vi "String add from start.vi"(4 "Datetime Format":enum16{"Full", "HH:MM:SS"}(ring), 5 "Display":bool=TRUE, 6 "Clear":bool, 7 "String Length":i32, 8 "error in (no error)":errorcluster, 10 "Main":string, 11 "Messages":refnum<vi>) -> (0 "error out":errorcluster, 3 "reference out":refnum<vi>)   [LabVIEW 2021]
doc: "为顶层UI的Message里面累计添加信息。最新的在最上面"
uses:
  <userlib>/John_Lib/DataBase/DataBase_SQL/DataBase_SQL.lvclass
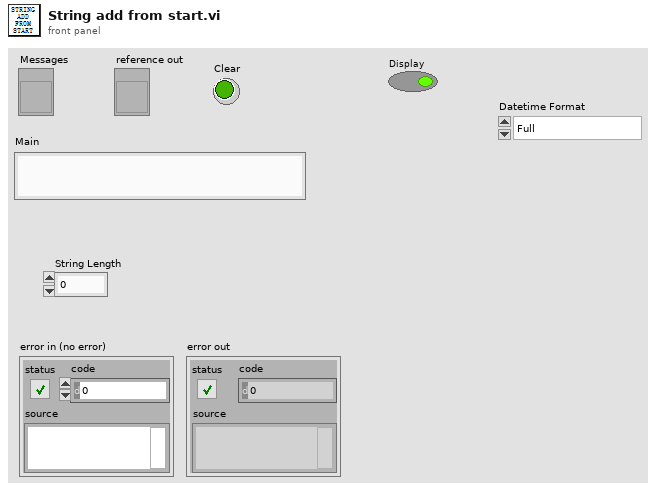
[diagram p1: front panel]
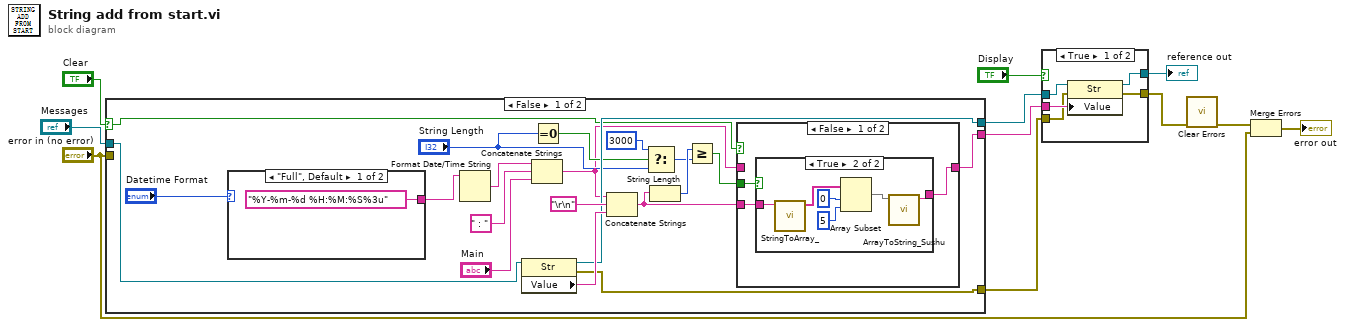
[diagram p0: block diagram]
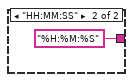
[diagram p3: hidden frame]
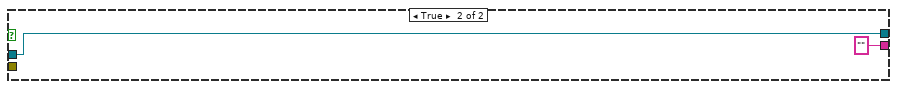
[diagram p6: hidden frame]
diagram:
  n1 = case shown="False" "Clear" {
    selector: "Clear" -> [w16 _]
    tunnel: "Messages" -> [w31 w46]
    tunnel: [w28 w46] -> w10
    tunnel: [w20 "" ("String")] -> w8
    tunnel: "error in (no error)" -> [_ _]
    tunnel: [w14 _] -> w5
    frame False {
      n2 = case shown="\"Full\", Default" "Datetime Format" {
        tunnel: ["%Y-%m-%d %H:%M:%S%3u" ("time format string (%c)") "%H:%M:%S" ("time format string (%c)")] -> w12
        frame "Full", Default {
        }
        frame "HH:MM:SS" {
        }
      }
      n3 = Format Date/Time String(time format string (%c)=w12) -> (date/time string=w27:string)  [unwired: 2 in]
      n4 = property class="Str"(reference=w31) -> (reference out=w28:refnum<vi>, error out=w14:errorcluster, "Value"=w29:string)  [unwired: 1 in]
      n5 = Concatenate Strings(w27, " : " ("string"), "Main") -> (w15:string)
      n6 = Equal To 0?(x="String Length") -> (x = 0?=w25:bool)
      n7 = Concatenate Strings(w15, "\r\n", w29) -> (w21:string)
      n8 = Select(t=3000 ("y"), s=w25, f="String Length") -> (s? t:f=w22:i32)
      n9 = String Length(string=w21) -> (length=w26:i32)
      n10 = Greater Or Equal?(x=w26, y=w22) -> (x >= y?=w17:bool)
      n11 = case shown="False" w16 {
        tunnel: w21 -> [w36 _]
        tunnel: [w35 w44] -> w20
        tunnel: w17 -> [w34 _]
        tunnel: w15 -> [_ w44]
        frame False {
          n12 = case shown="True" w34 {
            tunnel: w36 -> [w37 w41]
            tunnel: [w37 w38] -> w35
            frame False {
            }
            frame True {
              n13 = call <userlib>:"StringToArray_.vi"("State Queue"=w41) -> ("Array"=w40:string[])  [unwired: 7 in, 3 out]
              n14 = Array Subset(array=w40, index=0, length=5) -> (w39:string[])
              n15 = call <userlib>:"ArrayToString_Sushu.vi"("Array"=w39) -> ("String"=w38:string)  [unwired: 10 in]
            }
          }
        }
        frame True {
        }
      }
    }
    frame True {
    }
  }
  n16 = case shown="True" "Display" {
    tunnel: w10 -> [w51 w53]
    tunnel: [w50 w53] -> w9
    tunnel: w8 -> [w49 _]
    tunnel: w5 -> [w48 w52]
    tunnel: [w47 w52] -> w3
    frame True {
      n17 = property class="Str"(reference=w51, error in=w48, "Value"=w49) -> (reference out=w50:refnum<vi>, error out=w47:errorcluster)
    }
    frame False {
    }
  }
  "reference out" <- w9
  n18 = call <vilib>:"Clear Errors.vi"("error in (no error)"=w3) -> ("error out"=w2:errorcluster)  [unwired: 5 in, 1 out]
  n19 = Merge Errors(w2, "error in (no error)") -> (→"error out":errorcluster)
